vi "Remove Channel.vi"(7 "Channels Ctrl Ref":refnum<vi>, 8 "error in (no error)":errorcluster, 11 "To Save Wfm Arrays":waveform(dbl)[](array[waveform])) -> (0 "error out":errorcluster, 3 "Wfm Grp Data":T1)   [LabVIEW 2025, in "TDMS Waveform Creator UI.lvlib"]
uses:
  TDMS Waveform Creator UI.lvlib
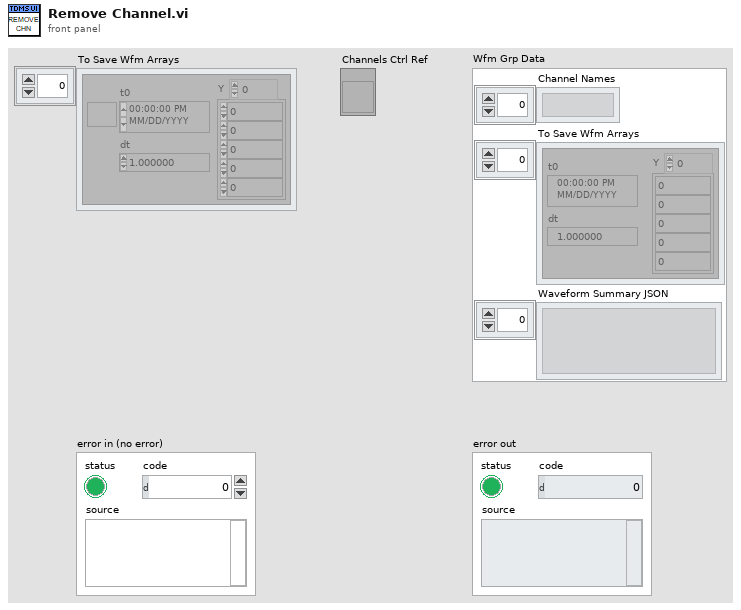
[diagram p1: front panel]
types:
  T1 = cluster{"Channel Names":string[], "To Save Wfm Arrays":waveform(dbl)[], "Waveform Summary JSON":string[]}
  T2 = cluster{"Item Names":string[], waveform(dbl)[], string[]}
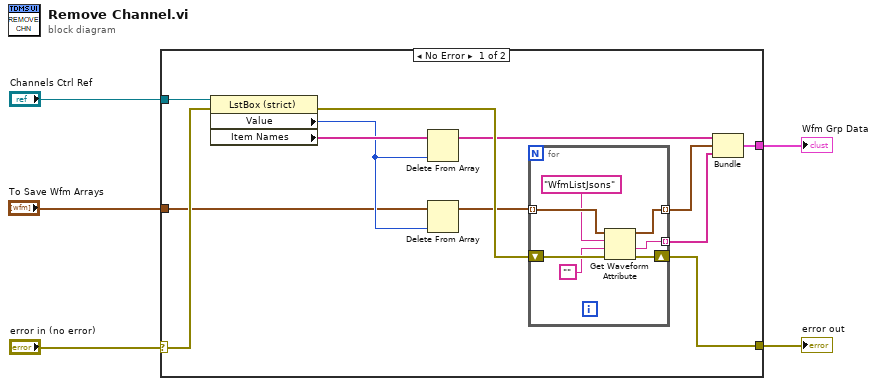
[diagram p0: block diagram]
diagram:
  n1 = case shown="No Error" "error in (no error)" {
    selector: "error in (no error)" -> [w16 w25]
    tunnel: "Channels Ctrl Ref" -> [w17 _]
    tunnel: "To Save Wfm Arrays" -> [w12 _]
    tunnel: [w10 w25] -> w2
    tunnel: [w6 _] -> w1
    frame No Error {
      n2 = property class="LstBox (strict)"(reference=w17, error in=w16) -> (error out=w15:errorcluster, "Value"=w13:i32, "Item Names"=w14:string[])  [unwired: 1 out]
      n3 = Delete From Array(array=w14, index=w13) -> (array with subset deleted=w9:string[])  [unwired: 1 in, 1 out]
      n4 = Delete From Array(array=w12, index=w13) -> (array with subset deleted=w11:waveform(dbl)[])  [unwired: 1 in, 1 out]
      n5 = for {
        shift-right: [w23] -> w10
        shift-left: w15 -> [w24]
        tunnel: w11 -> [w22] mode=indexing
        tunnel: [w21] -> w8 mode=indexing
        tunnel: [w18] -> w7 mode=indexing
        n6 = Get Waveform Attribute(4:w24, 5:"", 6:"WfmListJsons" ("name"), 7:w22) -> (0:w23:errorcluster, 1:w18:string, 3:w21:waveform(dbl))  [unwired: 1 out]
      }
      n7 = Bundle("Item Names"=w9, w8, w7) -> (w6:T2)  [unwired: 1 in]
    }
    frame Error {
    }
  }
  "error out" <- w2
  "Wfm Grp Data" <- w1
